vi "Set Report Orientation.vi"(0 "report in":refnum<class "NI_Standard Report.lvclass">, 5 "orientation (portrait)":i32(ring) items=["portrait", "landscape"], 11 "error in (no error)":errorcluster) -> (4 "report out":refnum<class "NI_Standard Report.lvclass">, 15 "error out":errorcluster)   [LabVIEW 2015, in "NI_Standard Report.lvclass"]
doc: "Determines whether the report is printed in landscape or portrait orientation."
uses:
  <vilib>/Utility/NIReport.llb/Standard Report/NI_Standard Report.lvclass
  <vilib>/Utility/NIReport.llb/Standard Report/NI_Standard Report.lvclass/NI_Standard Report.ctl
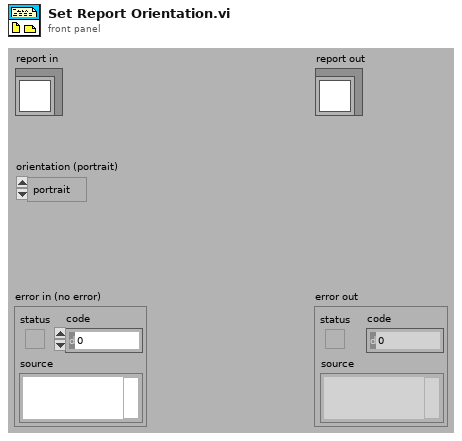
[diagram p1: front panel]
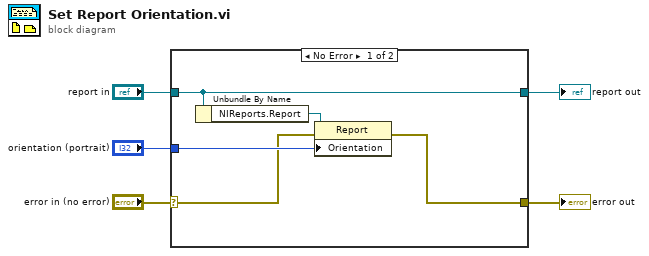
[diagram p0: block diagram]
diagram:
  n1 = case shown="No Error" "error in (no error)" {
    selector: "error in (no error)" -> [w7 w12]
    tunnel: [w6 w12] -> w4
    tunnel: [w9 w11] -> w2
    tunnel: "report in" -> [w9 w11]
    tunnel: "orientation (portrait)" -> [w8 _]
    frame No Error {
      n2 = Unbundle By Name(w9) -> ("NIReports.Report"=w10:refnum<k7>)
      n3 = property class="Report"(reference=w10, error in=w7, "Orientation"=w8) -> (error out=w6:errorcluster)  [unwired: 1 out]
    }
    frame Error {
    }
  }
  "error out" <- w4
  "report out" <- w2
